vi "AvaSpec Control.vi"(7 "Message Queue":refnum<queue>, 8 "error in (no error)":errorcluster, 9 "Path":path, 10 "Sphere Indicator":T2, 11 "VI in":refnum<vi>) -> (0 "error out":errorcluster, 3 "Color Parameters":T1)   [LabVIEW 2013]
uses:
  MeasurementControl Message Queue Folder/Message Cluster.ctl
  avantesSpectrometer/Acquisition/Sphere Indicator.ctl
  Color Parameters.ctl
  MeasurementControl Message Queue Folder/MeasurementControl Message Queue.lvlib
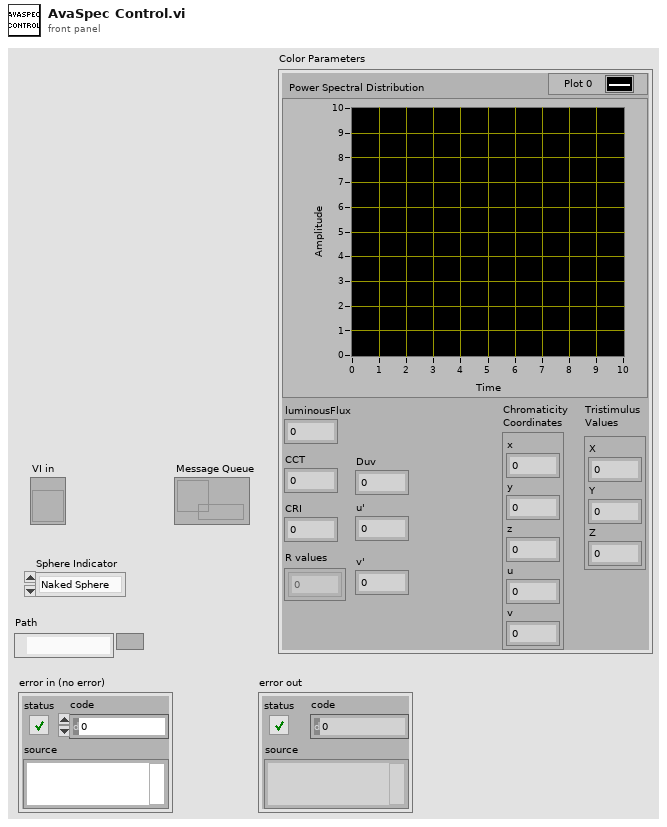
[diagram p1: front panel]
types:
  T1 = typedef "Color Parameters.ctl" = cluster{"Power Spectral Distribution":cluster{"X":dbl, "Y":dbl}[], "luminousFlux":dbl, "CCT":dbl, "CRI":dbl, "R values":dbl[], "Duv":dbl, "u'":dbl, "v'":dbl, "Chromaticity \nCoordinates":cluster{"x":dbl, "y":dbl, "z":dbl, "u":dbl, "v":dbl}, "Tristimulus \nValues":cluster{"X":dbl, "Y":dbl, "Z":dbl}}
  T2 = typedef "Sphere Indicator.ctl" = enum16{"Naked Sphere", "Insulated Sphere"}
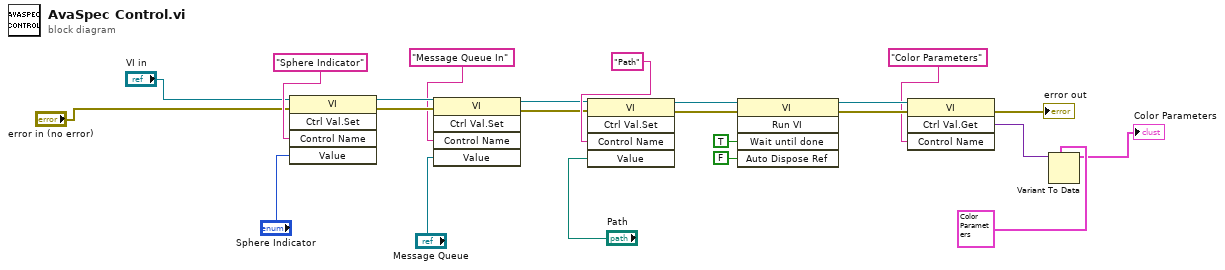
[diagram p0: block diagram]
diagram:
  n1 = invoke class="VI" method="Ctrl Val.Set"(reference="VI in", error in="error in (no error)", "Control Name"="Sphere Indicator", "Value"="Sphere Indicator") -> (reference out=w21:refnum<vi>, error out=w22:errorcluster)  [unwired: 1 in, 3 out]
  n2 = invoke class="VI" method="Ctrl Val.Set"(reference=w21, error in=w22, "Control Name"="Message Queue In", "Value"="Message Queue") -> (reference out=w19:refnum<vi>, error out=w20:errorcluster)  [unwired: 1 in, 3 out]
  n3 = invoke class="VI" method="Ctrl Val.Set"(reference=w19, error in=w20, "Control Name"="Path", "Value"="Path") -> (reference out=w18:refnum<vi>, error out=w8:errorcluster)  [unwired: 1 in, 3 out]
  n4 = invoke class="VI" method="Run VI"(reference=w18, error in=w8, "Wait until done"=TRUE ("Wait Until Done"), "Auto Dispose Ref"=FALSE ("Auto Dispose Reference")) -> (reference out=w17:refnum<vi>, error out=w7:errorcluster)  [unwired: 1 in, 3 out]
  n5 = invoke class="VI" method="Ctrl Val.Get"(reference=w17, error in=w7, "Control Name"="Color Parameters") -> (error out=→"error out":errorcluster, "Get Control Value Variant"=w5:variant)  [unwired: 1 in, 2 out]
  n6 = Variant To Data(type=T1 {"Power Spectral Distribution"=[], "luminousFlux"=0.0, "CCT"=0.0, "CRI"=0.0, "R values"=[], "Duv"=0.0, "u'"=0.0, "v'"=0.0, "Chromaticity \nCoordinates"={"x"=0.0, "y"=0.0, "z"=0.0, "u"=0.0, "v"=0.0}, "Tristimulus \nValues"={"X"=0.0, "Y"=0.0, "Z"=0.0}} ("Color Parameters"), Variant=w5) -> (data=→"Color Parameters":T1)  [unwired: 1 in, 1 out]
